vi "Shutdown.vi"(8 "error in (no error)":errorcluster, 11 "MockTransceiver in":refnum<class "MockTransceiver.lvclass">) -> (0 "error out":errorcluster, 3 "MockTransceiver out":refnum<class "MockTransceiver.lvclass">)   [LabVIEW 2017, in "MockTransceiver.lvclass"]
uses:
  MockTransceiver.lvclass
  MockTransceiver.lvclass/MockTransceiver.ctl
  Engine/Classes/Transceiver/Transceiver.lvclass
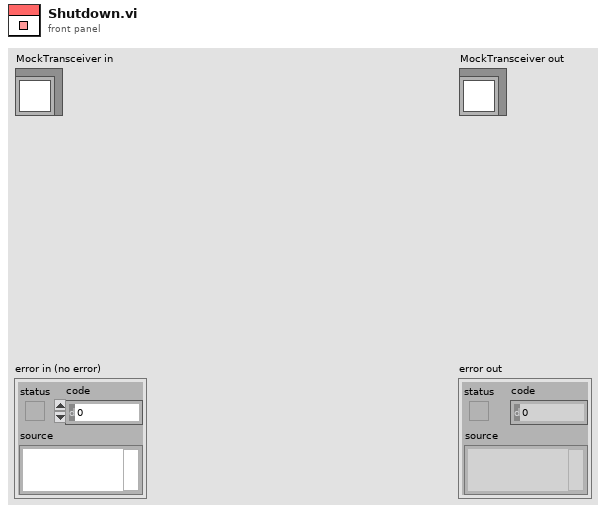
[diagram p1: front panel]
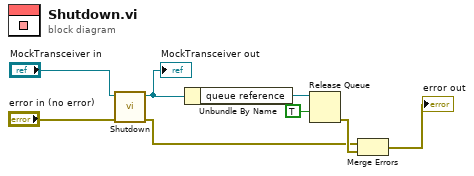
[diagram p0: block diagram]
diagram:
  n1 = call-parent "Shutdown.vi"("error in (no error)"="error in (no error)", "Transceiver in"="MockTransceiver in") -> ("error out"=w1:errorcluster, "Transceiver out"=w2:refnum<class "MockTransceiver.lvclass">)  [unwired: 8 in]
  "MockTransceiver out" <- w2
  n2 = Unbundle By Name(w2) -> ("queue reference"=w6:refnum<queue>)
  n3 = Release Queue(queue=w6, force destroy? (F)=TRUE) -> (error out=w5:errorcluster)  [unwired: 1 in, 2 out]
  n4 = Merge Errors(w1, w5) -> (→"error out":errorcluster)
